vi "Publish (Async).vi"(0 "WAMP Client in":refnum<class "WAMP Client.lvclass">, 5 "error in (no error)":errorcluster, 7 "Topic":string, 9 "Arguments":variant[](array[variant]), 11 "ArgumentsKw":string, 12 "Request Ack.":bool) -> (4 "WAMP Client out":refnum<class "WAMP Client.lvclass">, 6 "error out":errorcluster, 10 "Publish Results Event":refnum<user-event>)   [LabVIEW 2020, in "WAMP Client.lvclass"]
uses:
  <userlib>/lvwamp/WAMP Client/WAMP Client.lvclass
  <userlib>/lvwamp/WAMP Client/TypeDef/PUBLISH Result.ctl
  <userlib>/lvwamp/WAMP Client/TypeDef/Internal Message Type.ctl
  <userlib>/lvwamp/WAMP Client/TypeDef/PUBLISH Request Data.ctl
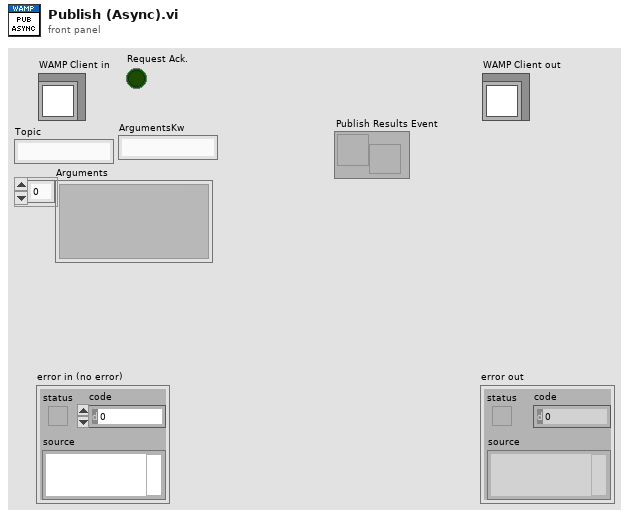
[diagram p1: front panel]
types:
  T1 = typedef "WAMP Client.lvclass/PUBLISH Request Data.ctl" = cluster{"Topic URI":string, "Arguments":variant[], "ArgumentsKw":string, "Publish Result Event":refnum<user-event>, "Request Ackoweldegemtn":bool}
  T2 = typedef "WAMP Client.lvclass/PUBLISH Result.ctl" = cluster{"Publish Request ID":u32, "Publication ID":u32, "Error":errorcluster, "Success?":bool}
  T3 = typedef "WAMP Client.lvclass/Internal Message Type.ctl" = enum16{"Subscribe", "Handle Subscribed", "Handle Event", "Unsubscribe", "Handle Unsubscribed", "Publish", "Handled Published", "Goodbye", "Handle Goodbye", "Call", "Handle Result"}
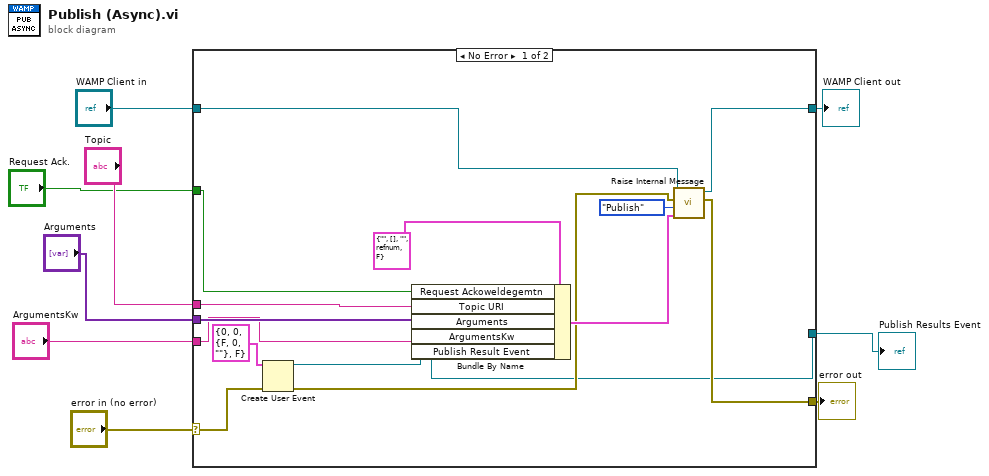
[diagram p0: block diagram]
diagram:
  n1 = case shown="No Error" "error in (no error)" {
    selector: "error in (no error)" -> [w17 w25]
    tunnel: [w15 w25] -> w8
    tunnel: [w14 w24] -> w6
    tunnel: "WAMP Client in" -> [w23 w24]
    tunnel: "Topic" -> [w21 _]
    tunnel: "Arguments" -> [w13 _]
    tunnel: "ArgumentsKw" -> [w12 _]
    tunnel: [w11 _] -> w2
    tunnel: "Request Ack." -> [w10 _]
    frame No Error {
      n2 = Create User Event(user event datatype=T2 {"Publish Request ID"=0, "Publication ID"=0, "Error"={"status"=FALSE, "code"=0, "source"=""}, "Success?"=FALSE} ("Cluster"), error in=w17) -> (user event=w11:refnum<user-event>, error out=w16:errorcluster)
      n3 = Bundle By Name(cluster=T1 {"Topic URI"="", "Arguments"=[], "ArgumentsKw"="", "Publish Result Event"=refnum, "Request Ackoweldegemtn"=FALSE} ("Cluster"), "Request Ackoweldegemtn"=w10, "Topic URI"=w21, "Arguments"=w13, "ArgumentsKw"=w12, "Publish Result Event"=w11) -> (w22:T1)
      n4 = call-dynamic "Raise Internal Message.vi"("Variant"=w22, "Internal Message Type"=Internal_Message_Type."Publish", "error in (no error)"=w16, "WAMP Client in"=w23) -> ("error out"=w15:errorcluster, "WAMP Client out"=w14:refnum<class "WAMP Client.lvclass">)  [unwired: 6 in]
    }
    frame Error {
    }
  }
  "error out" <- w8
  "WAMP Client out" <- w6
  "Publish Results Event" <- w2
